vi "Write Daq Channel Info.vi"(8 "error in (no error)":errorcluster, 10 "Daq Channel Info":T1, 11 "IODevConfig in":refnum<class "IODevConfig.lvclass">) -> (0 "error out":errorcluster, 3 "IODevConfig out":refnum<class "IODevConfig.lvclass">)   [LabVIEW 2015, in "IODevConfig.lvclass"]
uses:
  IODevConfig.lvclass
  Sequencer/Sequencer/Daq Channel Info.ctl
  IODevConfig.lvclass/IODevConfig.ctl
  Sequencer/Sequencer/Sequencer.lvclass
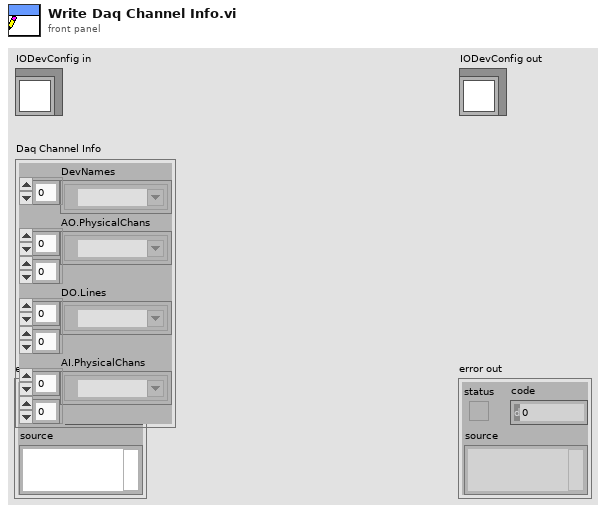
[diagram p1: front panel]
types:
  T1 = typedef "Sequencer.lvlib/Sequencer.lvclass/Daq Channel Info.ctl" = cluster{"DevNames":tag[], "AO.PhysicalChans":tag[][], "DO.Lines":tag[][], "AI.PhysicalChans":tag[][]}
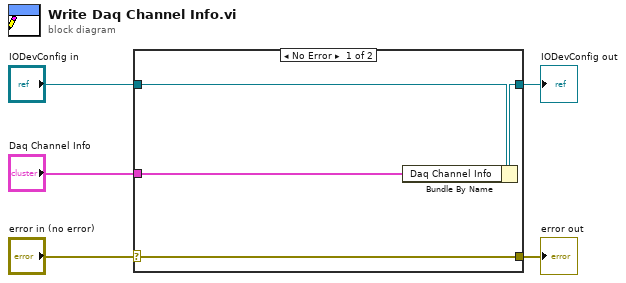
[diagram p0: block diagram]
diagram:
  n1 = case shown="No Error" "error in (no error)" {
    selector: "error in (no error)" -> [w9 w10]
    tunnel: [w9 w10] -> w4
    tunnel: [w7 w11] -> w2
    tunnel: "IODevConfig in" -> [w8 w11]
    tunnel: "Daq Channel Info" -> [w6 _]
    frame No Error {
      n2 = Bundle By Name(cluster=w8, "Daq Channel Info"=w6) -> (w7:refnum<class "IODevConfig.lvclass">)
    }
    frame Error {
    }
  }
  "error out" <- w4
  "IODevConfig out" <- w2
